vi "LinearFilter_BackwardFiniteDifference.vi"(9 "Period":dbl=0.02, 10 "Samples":i32, 11 "Derivative":i32) -> (0 "Error":bool, 3 "LINEAR_FILTER":T1 {"Outputs" format="%13.5g"; "Inputs" format="%13.5g"; "OutputGains" format="%13.5g"; "InputGains" format="%13.5g"})   [LabVIEW 2019, in "Trajectory_Library.lvlib"]
doc: "Creates a backward finite difference filter that computes the nth derivative of the input given the specified number of samples.\n \nFor example, a first derivative filter that uses two samples and a sample period of 20 ms would be\n \n LinearFilter_BackwardFiniteDifference(\n 1, \n 2, \n 0.02);\n\nFor additional information see:\n https://en.wikipedia.org/wiki/Finite_difference_coefficient#Arbitrary_stencil_points\n \nFor a given list of stencil points s of length n and the order of derivative d < n, the finite difference coefficients can be obtained by solving the following linear system for the vector a.\n\n [s1° ? s?° ][a1] [ d0,d ]\n [ ? ? ? ][? ] = d! [ ? ]\n [s1n?¹ ? s?n?¹][a?] [d??1,d]\n \n where d?,? are the Kronecker delta. The FIR gains are the elements of the\n vector a in reverse order divided by h?.\n \n The order of accuracy of the approximation is of the form O(hn??).\n\nInputs: \n - derivative -- The order of the derivative to compute.\n - samples -- The number of samples to use to compute the given derivative. This must be one more than the order of derivative or higher.\n - period -- The period in seconds between samples taken by the user.\n\nOutputs:\n - LINEAR FILTER - cluster containing:\n - InputGains - Array of “feedforward” or FIR gain factors (bx)\n - OutputGains - Array of “feedback” or IIR gain factors for feedback terms (ax)\n - Inputs - Array of the last n saved inputs\n - Outputs - Array of the last n saved outputs\n - InGainCount - Number of input gain terms\n - OutGainCount - number of output gain terms\n - Error -- Returns TRUE if an error occured."
uses:
  Trajectory_Library.lvlib
  TypeDef/LINEAR_FILTER.ctl
  Matrix_Create.vi
  LinearFilter_Factorial.vi
  LinearFilter_New.vi
  MatBuilder_Create.vi
  <vilib>/gmath/SpecialFunctions.llb/Factorial.vi
  <vilib>/Rock Robotics/SystemInterfaces/NetworkCommunication/NetComm_UsageReport_report.vi
  <vilib>/Analysis/7linalg.llb/Solve Linear Equations.vi
  <vilib>/Analysis/7linalg.llb/Solve Linear Equations (multiple right hand).vi
  Globals/Util_LibraryGlobals.vi
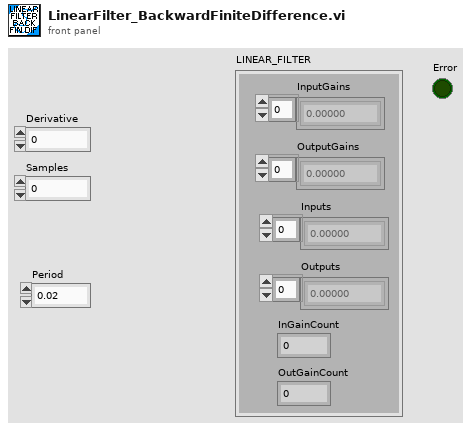
[diagram p1: front panel]
types:
  T1 = typedef "Trajectory_Library.lvlib/LINEAR_FILTER.ctl" = cluster{"InputGains":dbl[], "OutputGains":dbl[], "Inputs":dbl[], "Outputs":dbl[], "InGainCount":i32, "OutGainCount":i32}
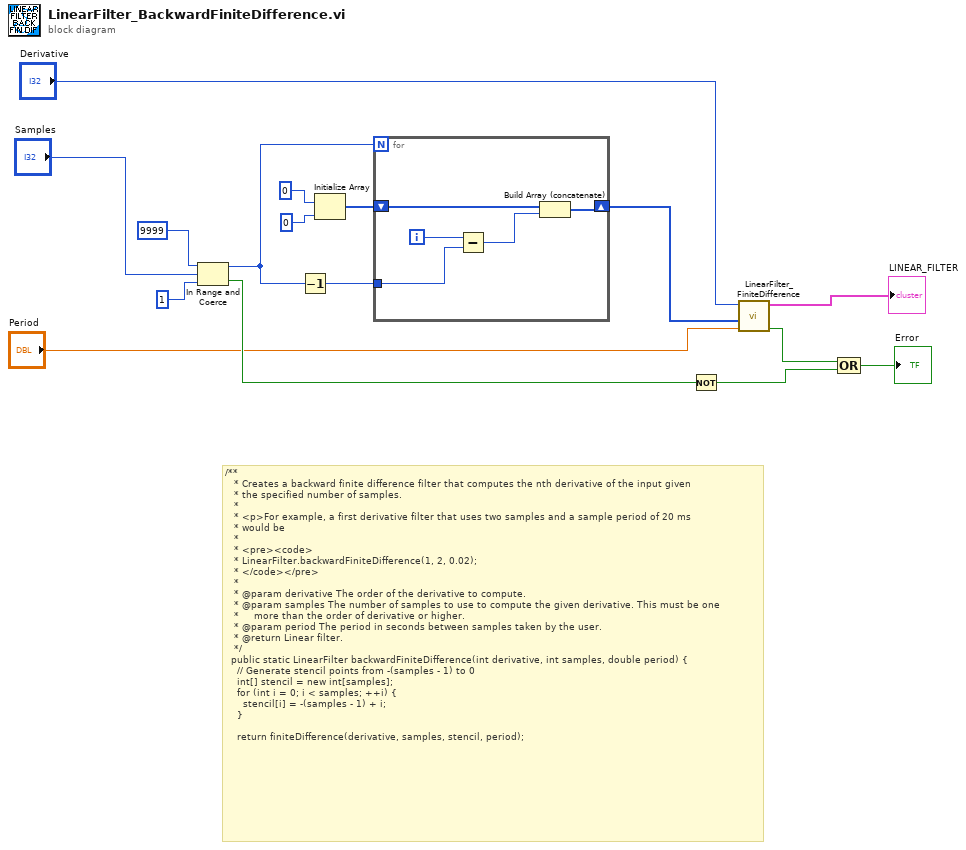
[diagram p0: block diagram]
diagram:
  # "/**\n   * Creates a backward finite difference filter that computes the nth derivative of the input given\n   * the specified number of samples.\n   *\n   * <p>For example, a first derivative filter that uses two samples and a sample period of 20 ms\n   * would be\n   *\n   * <pre><code>\n   * LinearFilter.backwardFiniteDifference(1, 2, 0.02);\n   * </code></pre>\n   *\n   * @param derivative The order of the derivative to compute.\n   * @param samples The number of samples to use to compute the given derivative. This must be one\n   *     more than the order of derivative or higher.\n   * @param period The period in seconds between samples taken by the user.\n   * @return Linear filter.\n   */\n  public static LinearFilter backwardFiniteDifference(int derivative, int samples, double period) {\n    // Generate stencil points from -(samples - 1) to 0\n    int[] stencil = new int[samples];\n    for (int i = 0; i < samples; ++i) {\n      stencil[i] = -(samples - 1) + i;\n    }\n\n    return finiteDifference(derivative, samples, stencil, period);"
  n1 = In Range and Coerce(upper limit=9999, x="Samples", lower limit=1) -> (coerced(x)=w8:i32, In Range?=w14:bool)
  n2 = Decrement(x=w8) -> (x-1=w7:i32)
  n3 = Initialize Array(0, 0 ("dimension size")) -> (w9:i32[])
  n4 = for {
    N: w8 -> [_]
    shift-right: [w20] -> w2
    shift-left: w9 -> [w21]
    tunnel: w7 -> [w18]
    i -> [w19]
    n5 = Subtract(x=w19, y=w18) -> (x-y=w17:i32)
    n6 = Build Array (concatenate)(w21, w17) -> (w20:i32[])
  }
  n7 = Not(x=w14) -> (.not. x?=w13:bool)
  n8 = call "LinearFilter_FiniteDifference.vi"("Period"="Period", "Stencil"=w2, "Derivative"="Derivative") -> ("Error"=w6:bool, "LINEAR_FILTER"=→"LINEAR_FILTER":T1)  [unwired: 7 in]
  n9 = Compound Arithmetic op=OR(w6, w13) -> (→"Error":bool)
